vi "Presa = Pnom.vi"(6 "RPM nom":dbl, 8 "C max freno [n/m]":dbl=2120.0, 9 "P imp (kw)":dbl) -> (1 "C [Nm]":dbl, 3 "C out%":dbl)   [LabVIEW 2019]
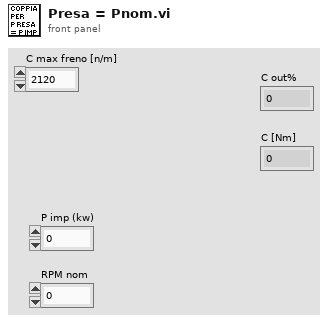
[diagram p1: front panel]
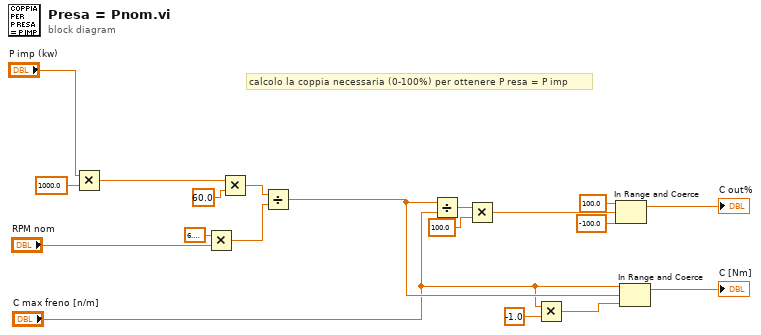
[diagram p0: block diagram]
diagram:
  # "calcolo la coppia necessaria (0-100%) per ottenere P resa = P imp"
  n1 = Multiply(x="P imp (kw)", y=1000.0) -> (x*y=w13:dbl)
  n2 = Multiply(x=6.283185307179586, y="RPM nom") -> (x*y=w18:dbl)
  n3 = Multiply(x=w13, y=60.0) -> (x*y=w17:dbl)
  n4 = Divide(x=w17, y=w18) -> (x/y=w5:dbl)
  n5 = Divide(x=w5, y="C max freno [n/m]") -> (x/y=w9:dbl)
  n6 = Multiply(x=w9, y=100.0) -> (x*y=w7:dbl)
  n7 = Multiply(x="C max freno [n/m]", y=-1.0) -> (x*y=w2:dbl)
  n8 = In Range and Coerce(upper limit=100.0, x=w7, lower limit=-100.0) -> (coerced(x)=→"C out%":dbl)  [unwired: 1 out]
  n9 = In Range and Coerce(upper limit="C max freno [n/m]", x=w5, lower limit=w2) -> (coerced(x)=→"C [Nm]":dbl)  [unwired: 1 out]
